vi "Get VI Image.vi"(8 "error in (no error)":errorcluster, 11 "VI Ref":refnum<vi>) -> (0 "error out":errorcluster, 2 "VI Image Data":T1, 3 "VI Ref out":refnum<vi>)   [LabVIEW 2020, in "MacroAssert.lvlib"]
doc: "Gets the VI image of the VI identified by <B>VI Ref</B>, and takes a subset of that image, the area determined by <B>subset rect</B>."
uses:
  MacroAssert.lvlib
  <vilib>/picture/picture.llb/imagedata.ctl
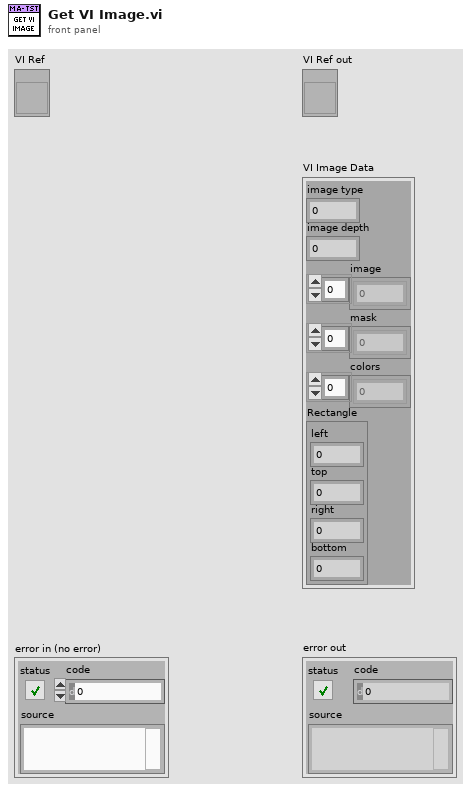
[diagram p1: front panel]
types:
  T1 = typedef "imagedata.ctl" = cluster{"image type":i32, "image depth":i32, "image":u8[], "mask":u8[], "colors":u32[], "Rectangle":cluster{"left":i16, "top":i16, "right":i16, "bottom":i16}}
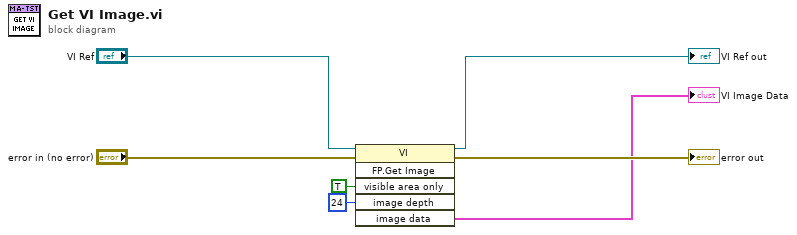
[diagram p0: block diagram]
diagram:
  n1 = invoke class="VI" method="FP.Get Image"(reference="VI Ref", error in="error in (no error)", "visible area only"=TRUE ("Visible Area Only"), "image depth"=24 ("Image Depth")) -> (reference out=→"VI Ref out":refnum<vi>, error out=→"error out":errorcluster, "image data"=→"VI Image Data":T1)  [unwired: 2 in, 3 out]
